vi "_DegreesToRadians.vi"(9 "Degrees In":dbl) -> (10 "Radians":dbl)   [LabVIEW 2023]
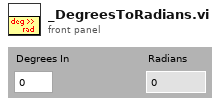
[diagram p1: front panel]
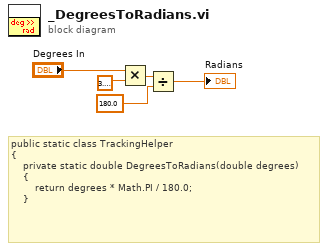
[diagram p0: block diagram]
diagram:
  # "public static class TrackingHelper\n{\n    private static double DegreesToRadians(double degrees)\n    {\n        return degrees * Math.PI / 180.0;\n    }"
  n1 = Multiply(x="Degrees In", y=3.141592653589793) -> (x*y=w3:dbl)
  n2 = Divide(x=w3, y=180.0) -> (x/y=→"Radians":dbl)
